vi "New SSL Client Socket Hostname.vi"(6 "Verify hostname? (T)":bool=TRUE, 8 "error in (no error)":errorcluster, 9 "timeout ms (5000)":i32=5000, 10 "Hostname / URL":string="echo.websocket.org:443", 11 "SSL Client Ctx":refnum<class "SSL Client Context.lvclass">) -> (0 "error out":errorcluster, 3 "SSL Client Skt out":refnum<class "SSL Client Socket.lvclass">)   [LabVIEW 2013]
doc: "Creates a new SSL Client Socket and connects to the server."
uses:
  SSL Client Socket.lvclass
  SSL Client Context/SSL Client Context.lvclass
  <vilib>/MediaMongrels Ltd/WebSockets/WebSockets/WebSocket Client/WebSocket Client.lvclass
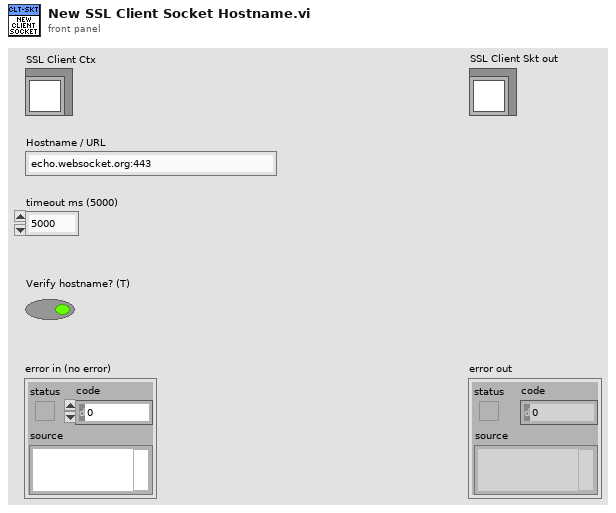
[diagram p1: front panel]
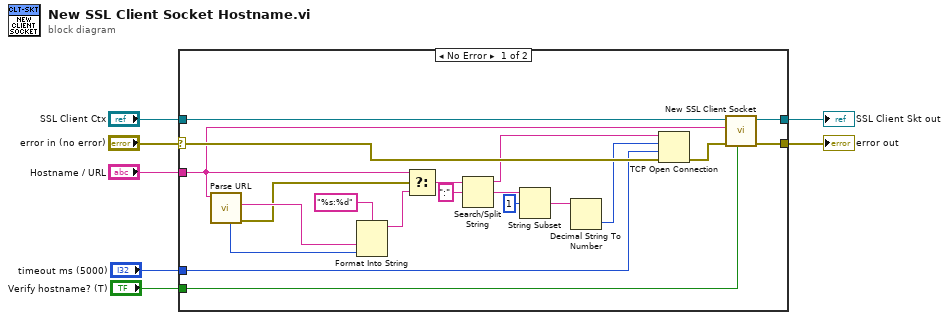
[diagram p0: block diagram]
diagram:
  n1 = case shown="No Error" "error in (no error)" {
    selector: "error in (no error)" -> [w18 w28]
    tunnel: [w27 w28] -> w6
    tunnel: "SSL Client Ctx" -> [w25 _]
    tunnel: "Hostname / URL" -> [w8 _]
    tunnel: [w26 _] -> w3
    tunnel: "Verify hostname? (T)" -> [w24 _]
    tunnel: "timeout ms (5000)" -> [w9 _]
    frame No Error {
      n2 = call <vilib>:"Parse URL.vi"("WebSocket URL"=w8) -> ("error out"=w20:errorcluster, "host"=w23:string, "port"=w22:u16)  [unwired: 6 in, 2 out]
      n3 = Format Into String(format string="%s:%d", w23, w22) -> (resulting string=w19:string)  [unwired: 2 in, 1 out]
      n4 = Select(t=w8, s=w20, f=w19) -> (s? t:f=w16:string)
      n5 = Search/Split String(string=w16, search string/char (-)=":") -> (substring before match=w12:string, match + rest of string=w14:string)  [unwired: 1 in, 1 out]
      n6 = String Subset(string=w14, offset (0)=1) -> (substring=w11:string)  [unwired: 1 in]
      n7 = Decimal String To Number(string=w11) -> (number=w10:i32)  [unwired: 2 in, 1 out]
      n8 = TCP Open Connection(address=w12, remote port or service name=w10, timeout ms (60000)=w9, error in (no error)=w18) -> (error out=w17:errorcluster)  [unwired: 1 in, 1 out]
      n9 = call "New SSL Client Socket.vi"("Verify hostname? (T)"=w24, "error in (no error)"=w17, "Hostname / URL"=w8, "SSL Client Ctx"=w25) -> ("error out"=w27:errorcluster, "SSL Client Skt out"=w26:refnum<class "SSL Client Socket.lvclass">)  [unwired: 6 in]
    }
    frame Error {
    }
  }
  "error out" <- w6
  "SSL Client Skt out" <- w3
